vi "CCD bias dependent spectrum.vi"() -> ()   [LabVIEW 2012]
uses:
  <vilib>/Utility/file.llb/Read From Spreadsheet File (DBL).vi
  Instance           3 35Saved   CCD photon image_540_800_CR .vi
  Instance           4 35Saved   CCD photon image_540_800_CR .vi
  Instance           5 35Saved   CCD photon image_540_800_CR .vi
  Instance           8 35Saved   CCD photon image_540_800_CR .vi
  Instance          12 35Saved   CCD photon image_540_800_CR .vi
panel:
  in  "offset":dbl
  in  "gain":dbl=1.0
  out "Window 2":cluster{"Y":dbl[], "Y":dbl[]}[](graph)
  out "Window 1":cluster{"Y":dbl[], "Y":dbl[]}[](graph)
  in  "bias to":dbl=950.0
  in  "Bias from":dbl=550.0
  in  "Full Range":bool
  in  "Full Range":bool
  out "Save As":string
  in  "Save Matrix2":bool
  out "Save As":string
  in  "Save Matrix1":bool
  in  "select 2":bool
  in  "select":bool
  in  "next 2":bool
  in  "next":bool
  in  "previous 2":bool
  in  "previous":bool
  in  "Do it":bool
  out "?":path
  out "?":path
  out "pixnum":i32
  in  "?":bool
  in  "stop 2":bool
  in  "spc to":dbl=950.0
  in  "Spc From":dbl=550.0
  in  "?":bool
  out "MAX":dbl
  out "MIN":dbl
  out "X":sgl
  out "Y":sgl
  out "px":dbl
  out "px":dbl
  out "eV":dbl format="%#_4g"
  out "eV":dbl format="%#_4g"
  in  "To":dbl
  in  "From":dbl
  out "spc size":dbl=32.0
  out "eV":dbl format="%#_4g"
  out "eV":dbl format="%#_4g"
  in  "To":dbl
  in  "From":dbl
  out "px":dbl
  out "px":dbl
  in  "#2":bool
  # "Input File"
  # "2 Files"
  # "1 File"
  # "1st"
  # "2nd"
  # "Spectra Range"
  # "nm"
  # "to"
  # "nm"
  # "From"
  # "Bias Range"
  # "From"
  # "to"
  # "eV"
  # "eV"
  # "nm"
  # "# of Pixel"
  # "# of Spectra"
  # "nm"
  # "Offset"
  # "Gain"
  # "Active Window"
  # "#1"
  # "#2"
  # "Cosmic Ray Removal"
  # "NO"
  # "YES"
  # "Value"
  # "Position"
  # "nm"
  # "nm"
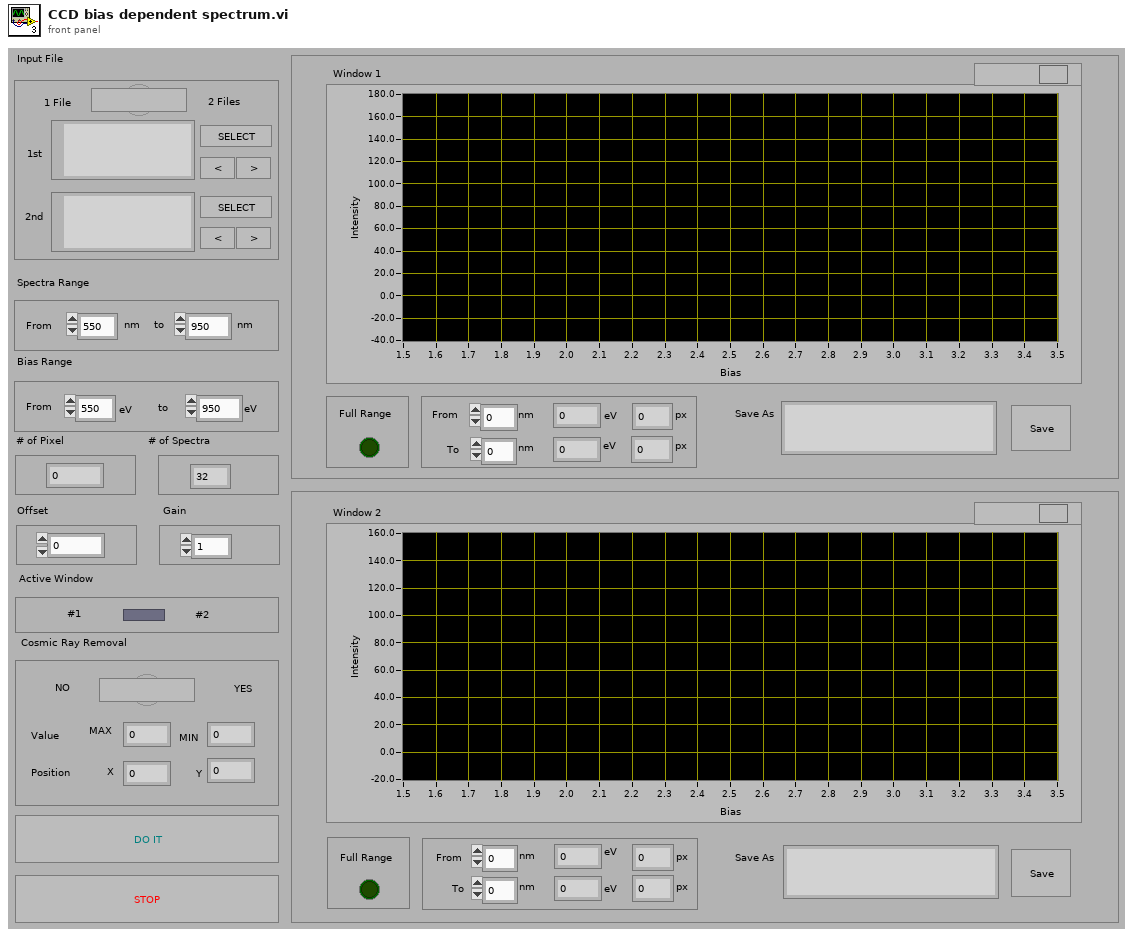
[diagram p1: front panel]
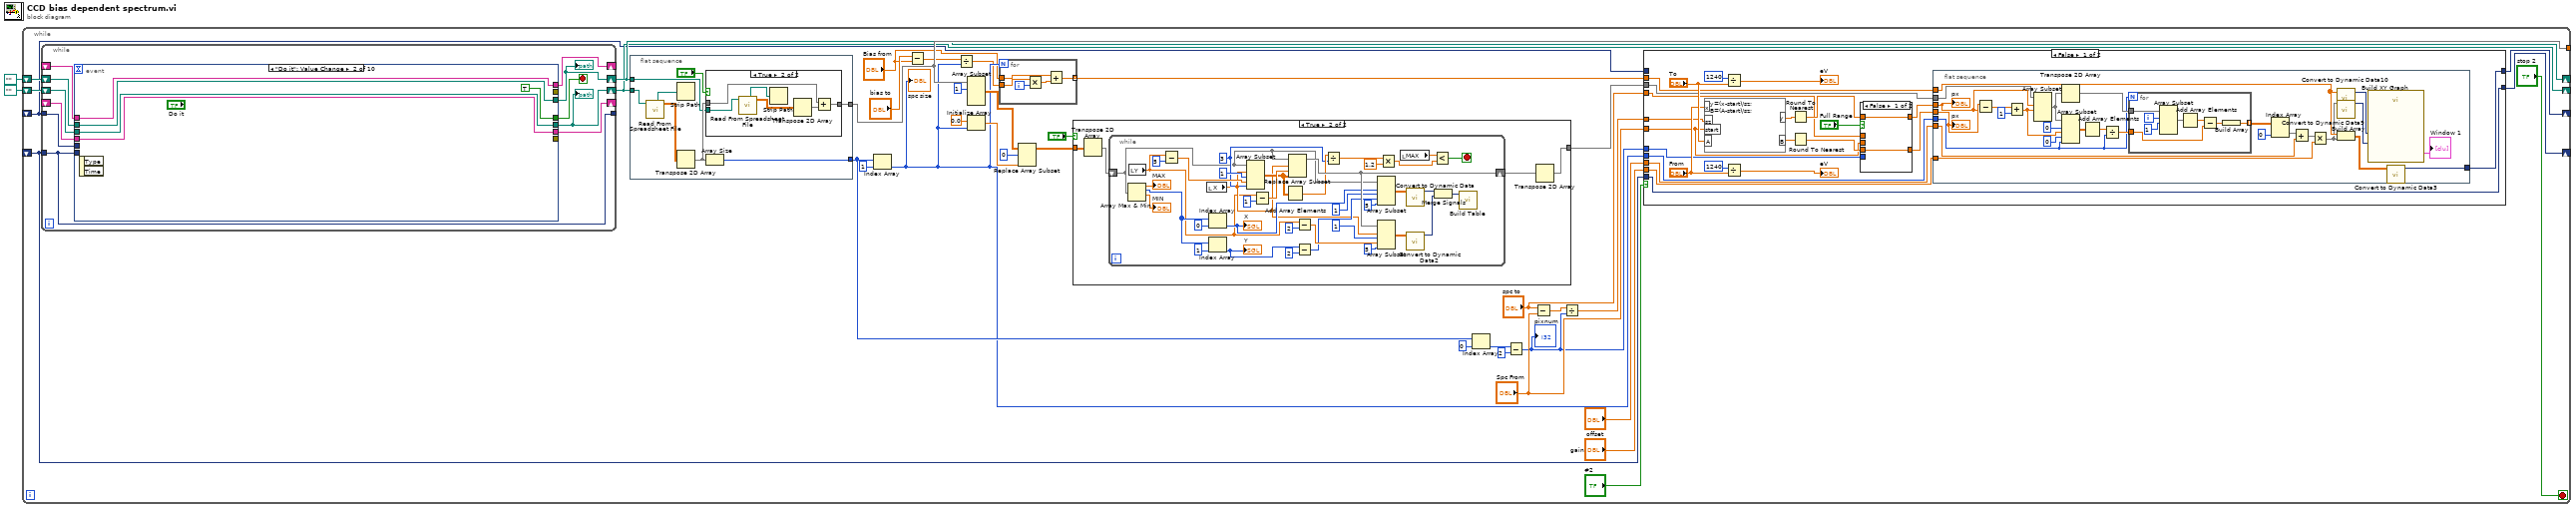
[diagram p0: block diagram]
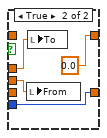
[diagram p2: hidden frame]
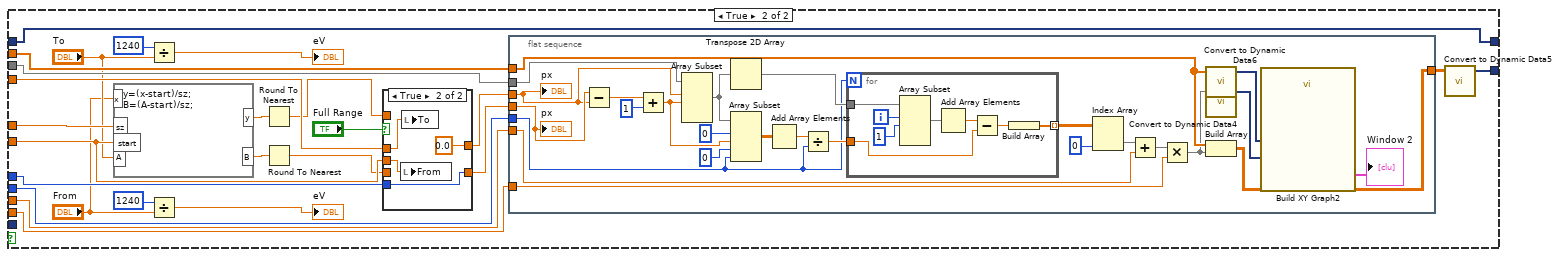
[diagram p3: hidden frame]
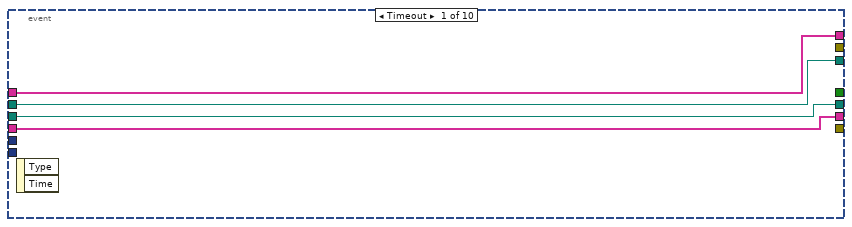
[diagram p5: hidden frame]
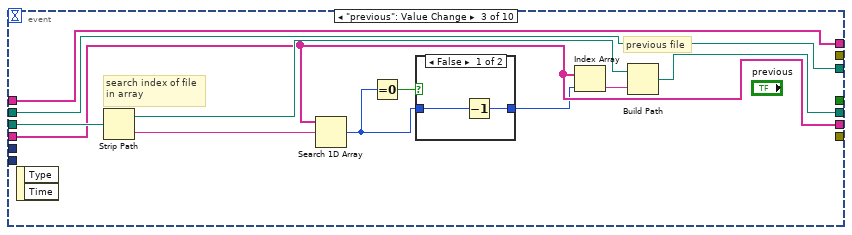
[diagram p6: hidden frame]
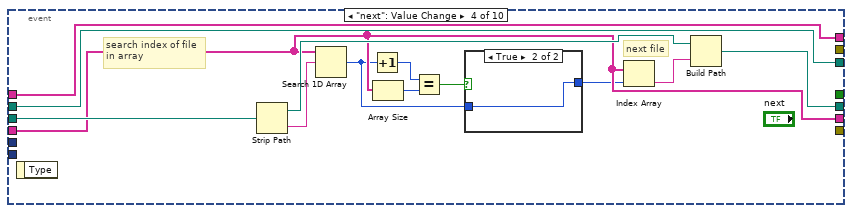
[diagram p8: hidden frame]
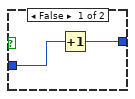
[diagram p9: hidden frame]
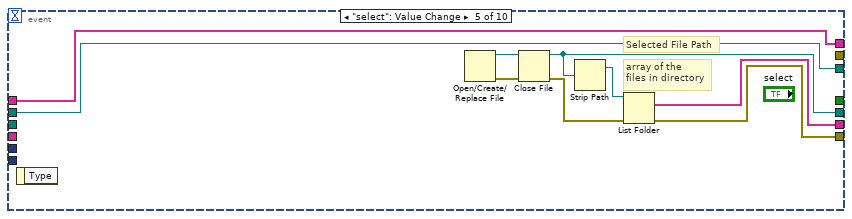
[diagram p10: hidden frame]
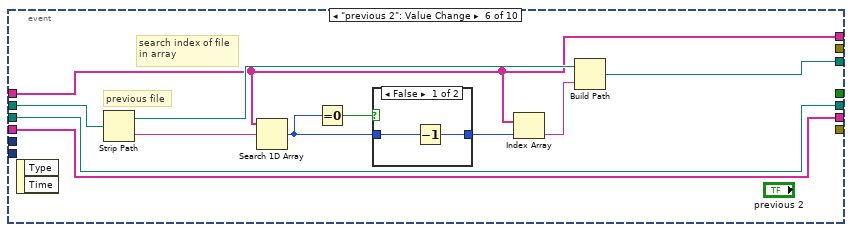
[diagram p11: hidden frame]
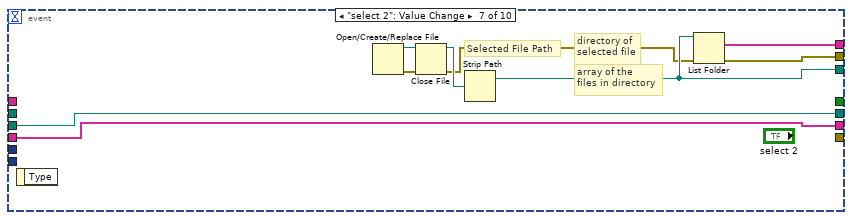
[diagram p13: hidden frame]
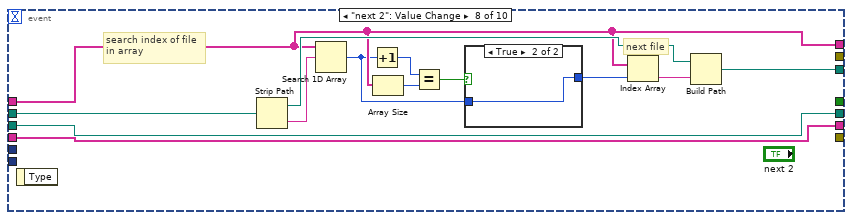
[diagram p14: hidden frame]
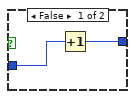
[diagram p15: hidden frame]
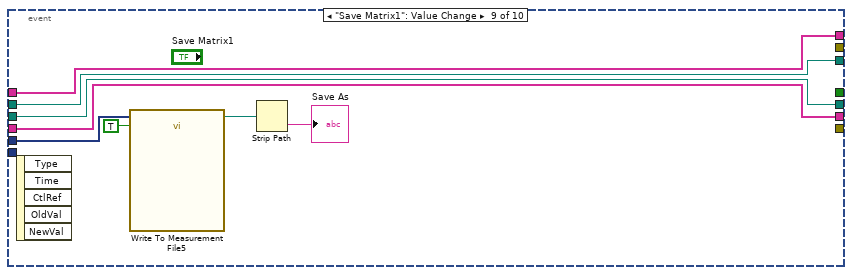
[diagram p16: hidden frame]
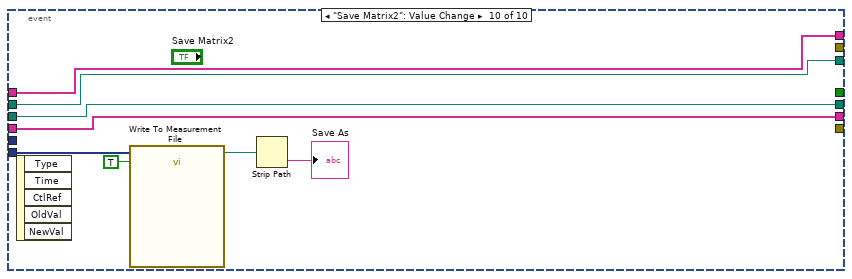
[diagram p17: hidden frame]
diagram:
  n1 = while {
    tunnel: [w27] -> _
    shift-right: [w20] -> _
    shift-left: path "" ("path") -> [w22]
    shift-right: [w21] -> _
    shift-left: path "" ("path") -> [w23]
    shift-right: [w19] -> _
    shift-left: _ -> [w5]
    shift-right: [w18] -> _
    shift-left: _ -> [w6]
    stop <- "stop 2" stop-if-true
    n2 = while {
      shift-right: [w185] -> _
      shift-left: _ -> [w184]
      shift-right: [w175] -> w20
      shift-left: w22 -> [w183]
      shift-right: [w176] -> w21
      shift-left: w23 -> [w182]
      shift-right: [w181] -> _
      shift-left: _ -> [w180]
      tunnel: w5 -> [w178]
      tunnel: w6 -> [w177]
      tunnel: [w177] -> _
      stop <- w179 stop-if-true
      n3 = event shown="[1] \"Do it\": Value Change" {
        selector: _ -> [_ _ _ _ _ _ _ _ _ _]
        dyn-events: _ -> [_ _ _ _ _ _ _ _ _ _]
        timeout: _ -> [_ _ _ _ _ _ _ _ _ _]
        tunnel: [_ TRUE _ _ _ _ _ _ _ _] -> w179
        tunnel: [w188 w193 w200 w218 w228 w234 w255 w264 w276 w282] -> w175
        tunnel: [w189 w194 w202 w214 w232 w239 w254 w263 w273 w281] -> w185
        tunnel: w184 -> [w189 w194 w202 w214 _ w239 w254 w263 w273 w281]
        tunnel: w183 -> [w188 w193 w205 w217 _ w234 w255 w264 w276 w282]
        tunnel: [w186 w191 w198 w215 w230 w235 w253 w265 w275 w283] -> w176
        tunnel: w182 -> [w186 w191 w198 w215 w230 w241 _ w266 w275 w283]
        tunnel: [w187 w192 w199 w216 w231 w240 w256 w259 w274 w284] -> w181
        tunnel: w180 -> [w187 w192 w199 w216 w231 w240 _ w259 w274 w284]
        tunnel: w178 -> [_ _ _ _ _ _ _ _ w280 _]
        tunnel: w177 -> [_ _ _ _ _ _ _ _ _ w288]
        tunnel: [_ _ _ _ _ _ w248 _ _ _] -> _
        tunnel: [_ _ _ _ w225 _ _ _ _ _] -> _
        event Timeout {
          n4 = event-data() -> ()  [unwired: 1 in, 2 out]
        }
        event "Do it": Value Change {
          n5 = event-data() -> ()  [unwired: 1 in, 2 out]
        }
        event "previous": Value Change {
          # "previous file"
          # "search index of file\nin array"
          n6 = event-data() -> ()  [unwired: 1 in, 2 out]
          n7 = Strip Path(path=w205) -> (stripped path=w203:path, name=w204:string)
          n8 = Search 1D Array(1D array=w202, element=w204) -> (index of element=w196:i32)  [unwired: 1 in]
          n9 = Equal To 0?(x=w196) -> (x = 0?=w197:bool)
          n10 = case shown="False" w197 {
            tunnel: w196 -> [w207 w208]
            tunnel: [w206 w208] -> w195
            frame False {
              n11 = Decrement(x=w207) -> (x-1=w206:i32)
            }
            frame True {
            }
          }
          n12 = Index Array(array=w202, index=w195) -> (element=w201:string)
          n13 = Build Path(base path=w203, name or relative path=w201) -> (appended path=w200:path)
        }
        event "next": Value Change {
          # "next file"
          # "search index of file\nin array"
          n14 = event-data() -> ()  [unwired: 1 in, 1 out]
          n15 = Strip Path(path=w217) -> (stripped path=w220:path, name=w221:string)
          n16 = Search 1D Array(1D array=w214, element=w221) -> (index of element=w209:i32)  [unwired: 1 in]
          n17 = Increment(x=w209) -> (x+1=w210:i32)
          n18 = Array Size(array=w214) -> (size(s)=w213:i32)
          n19 = Equal?(x=w210, y=w213) -> (x = y?=w212:bool)
          n20 = case shown="True" w212 {
            tunnel: w209 -> [w223 w224]
            tunnel: [w222 w224] -> w211
            frame False {
              n21 = Increment(x=w223) -> (x+1=w222:i32)
            }
            frame True {
            }
          }
          n22 = Index Array(array=w214, index=w211) -> (element=w219:string)
          n23 = Build Path(base path=w220, name or relative path=w219) -> (appended path=w218:path)
        }
        event "select": Value Change {
          # "array of the \nfiles in directory"
          # "Selected File Path"
          n24 = event-data() -> ()  [unwired: 1 in, 1 out]
          n25 = Open/Create/Replace File() -> (refnum out=w229:refnum<file>, error out=w227:errorcluster)  [unwired: 6 in, 1 out]
          n26 = Close File(refnum=w229, error in=w227) -> (path=w228:path, error out=w226:errorcluster)
          n27 = Strip Path(path=w228) -> (stripped path=w233:path)  [unwired: 1 out]
          n28 = List Folder(path=w233, error in=w226) -> (filenames=w232:string[], error out=w225:errorcluster)  [unwired: 2 in, 2 out]
        }
        event "previous 2": Value Change {
          # "previous file"
          # "search index of file\nin array"
          n29 = event-data() -> ()  [unwired: 1 in, 2 out]
          n30 = Strip Path(path=w241) -> (stripped path=w243:path, name=w244:string)
          n31 = Search 1D Array(1D array=w240, element=w244) -> (index of element=w237:i32)  [unwired: 1 in]
          n32 = Equal To 0?(x=w237) -> (x = 0?=w238:bool)
          n33 = case shown="False" w238 {
            tunnel: w237 -> [w246 w247]
            tunnel: [w245 w247] -> w236
            frame False {
              n34 = Decrement(x=w246) -> (x-1=w245:i32)
            }
            frame True {
            }
          }
          n35 = Index Array(array=w240, index=w236) -> (element=w242:string)
          n36 = Build Path(base path=w243, name or relative path=w242) -> (appended path=w235:path)
        }
        event "select 2": Value Change {
          # "array of the \nfiles in directory"
          # "directory of\nselected file"
          # "Selected File Path"
          n37 = event-data() -> ()  [unwired: 1 in, 1 out]
          n38 = Open/Create/Replace File() -> (refnum out=w252:refnum<file>, error out=w250:errorcluster)  [unwired: 6 in, 1 out]
          n39 = Close File(refnum=w252, error in=w250) -> (path=w251:path, error out=w249:errorcluster)
          n40 = Strip Path(path=w251) -> (stripped path=w253:path)  [unwired: 1 out]
          n41 = List Folder(path=w253, error in=w249) -> (filenames=w256:string[], error out=w248:errorcluster)  [unwired: 2 in, 2 out]
        }
        event "next 2": Value Change {
          # "next file"
          # "search index of file\nin array"
          n42 = event-data() -> ()  [unwired: 1 in, 1 out]
          n43 = Strip Path(path=w266) -> (stripped path=w268:path, name=w269:string)
          n44 = Search 1D Array(1D array=w259, element=w269) -> (index of element=w258:i32)  [unwired: 1 in]
          n45 = Increment(x=w258) -> (x+1=w260:i32)
          n46 = Array Size(array=w259) -> (size(s)=w262:i32)
          n47 = Equal?(x=w260, y=w262) -> (x = y?=w261:bool)
          n48 = case shown="True" w261 {
            tunnel: w258 -> [w271 w272]
            tunnel: [w270 w272] -> w257
            frame False {
              n49 = Increment(x=w271) -> (x+1=w270:i32)
            }
            frame True {
            }
          }
          n50 = Index Array(array=w259, index=w257) -> (element=w267:string)
          n51 = Build Path(base path=w268, name or relative path=w267) -> (appended path=w265:path)
        }
        event "Save Matrix1": Value Change {
          n52 = event-data() -> ()  [unwired: 1 in, 5 out]
          n53 = call "Write To Measurement File5"("Signals"=w280, "Reset"=TRUE) -> ("Filename Out"=w278:path)  [unwired: 15 in, 2 out]
          n54 = Strip Path(path=w278) -> (name=→"Save As":string)  [unwired: 1 out]
        }
        event "Save Matrix2": Value Change {
          n55 = event-data() -> ()  [unwired: 1 in, 5 out]
          n56 = call "Write To Measurement File"("Signals"=w288, "Reset"=TRUE) -> ("Filename Out"=w286:path)  [unwired: 15 in, 2 out]
          n57 = Strip Path(path=w286) -> (name=→"Save As":string)  [unwired: 1 out]
        }
      }
      "?" <- w175
      "?" <- w176
    }
    n58 = flat-sequence {
      tunnel: [w295] -> w27
      tunnel: [w292] -> w15
      tunnel: w20 -> [w290]
      tunnel: w21 -> [w289]
      frame #0 {
        n59 = call-poly <vilib>:"Read From Spreadsheet File.vi"("file path (dialog if empty)"=w290) -> ("all rows"=w293:dbl[][], "new file path (Not A Path if cancelled)"=w296:path)  [unwired: 6 in, 3 out]
        n60 = Strip Path(path=w296) -> ()  [unwired: 2 out]
        n61 = Transpose 2D Array(2D array=w293) -> (transposed array=w291:dbl[][])
        n62 = case shown="True" "?" {
          tunnel: w291 -> [w297 w302]
          tunnel: [w297 w301] -> w295
          tunnel: w289 -> [_ w298]
          frame False {
          }
          frame True {
            n63 = call-poly <vilib>:"Read From Spreadsheet File.vi"("file path (dialog if empty)"=w298) -> ("all rows"=w300:dbl[][], "new file path (Not A Path if cancelled)"=w303:path)  [unwired: 6 in, 3 out]
            n64 = Strip Path(path=w303) -> ()  [unwired: 2 out]
            n65 = Transpose 2D Array(2D array=w300) -> (transposed array=w299:dbl[][])
            n66 = Add(x=w302, y=w299) -> (x+y=w301:dbl[][])
          }
        }
        n67 = Array Size(array=w291) -> (size(s)=w292:i32[])
      }
    }
    n68 = Index Array(array=w15, index=1) -> (element=w11:i32)
    "spc size" <- w11
    n69 = Subtract(x="bias to", y="Bias from") -> (x-y=w12:dbl)
    n70 = Divide(x=w12, y=w11) -> (x/y=w10:dbl)
    n71 = Array Subset(array=w27, index (row)=1) -> (w36:dbl[][])  [unwired: 3 in]
    n72 = Initialize Array(0.0 ("element"), w11) -> (w38:dbl[])
    n73 = for {
      N: w11 -> [_]
      tunnel: [w170] -> w8 mode=indexing
      tunnel: w10 -> [w173]
      tunnel: "Bias from" -> [w171]
      i -> [w174]
      n74 = Multiply(x=w173, y=w174) -> (x*y=w172:dbl)
      n75 = Add(x=w171, y=w172) -> (x+y=w170:dbl)
    }
    n76 = Replace Array Subset(array=w36, new element=w38, index (row)=0) -> (w34:dbl[][])  [unwired: 1 in]
    n77 = case shown="True" "?" {
      tunnel: w34 -> [w304 w308]
      tunnel: [w304 w306] -> w33
      frame False {
      }
      frame True {
        n78 = Transpose 2D Array(2D array=w308) -> (transposed array=w307:dbl[][])
        n79 = while {
          shift-right: [w345] -> w305
          shift-left: w307 -> [w309]
          stop <- w324 stop-if-true
          w322 = 3
          n80 = Array Max & Min(array=w309) -> (max value=→"MAX":dbl, max index (indices)=w343:i32[], min value=→"MIN":dbl)  [unwired: 1 out]
          n81 = local read "Y"() -> (w311:sgl)
          n82 = Subtract(x=w311, y=5) -> (x-y=w339:sgl)
          n83 = local read "X"() -> (w312:sgl)
          n84 = Index Array(array=w343, index=0) -> (element=w316:i32)
          "X" <- w316
          n85 = Index Array(array=w343, index=1) -> (element=w315:i32)
          "Y" <- w315
          n86 = Array Subset(array=w309, index (row)=w312, length (row)=1, index (col)=w339, length (col)=w322) -> (w321:dbl[][])
          n87 = Subtract(x=w311, y=1) -> (x-y=w338:sgl)
          n88 = Add Array Elements(numeric array=w321) -> (sum=w323:dbl)
          n89 = Replace Array Subset(array=w309, new element=w321, index (row)=w312, index (col)=w338) -> (w345:dbl[][])
          n90 = Subtract(x=w311, y=2) -> (x-y=w334:sgl)
          n91 = Subtract(x=w315, y=2) -> (x-y=w329:i32)
          n92 = Divide(x=w323, y=w322) -> (x/y=w320:dbl)
          n93 = Array Subset(array=w309, index (row)=w316, length (row)=1, index (col)=w329, length (col)=5) -> (w327:dbl[][])
          n94 = Array Subset(array=w345, index (row)=w312, length (row)=1, index (col)=w334, length (col)=5) -> (w332:dbl[][])
          n95 = Multiply(x=w320, y=1.2) -> (x*y=w325:dbl)
          n96 = local read "MAX"() -> (w310:dbl)
          n97 = call "Convert to Dynamic Data"("2D Array"=w327) -> ("Dynamic Data Type"=w319:dynamicdata)  [unwired: 3 in]
          n98 = call "Convert to Dynamic Data2"("2D Array"=w332) -> ("Dynamic Data Type"=w317:dynamicdata)  [unwired: 3 in]
          n99 = Less?(x=w310, y=w325) -> (x < y?=w324:bool)
          n100 = Merge Signals(w319, w317) -> (w318:dynamicdata)
          n101 = call "Build Table"("Signals"=w318) -> ()  [unwired: 9 in, 2 out]
        }
        n102 = Transpose 2D Array(2D array=w305) -> (transposed array=w306:dbl[][])
      }
    }
    n103 = Index Array(array=w15, index=0) -> (element=w25:i32)
    n104 = Subtract(x=w25, y=2) -> (x-y=w17:i32)
    "pixnum" <- w17
    n105 = Subtract(x="spc to", y="Spc From") -> (x-y=w31:dbl)
    n106 = Divide(x=w31, y=w17) -> (x/y=w30:dbl)
    n107 = case shown="False" "#2" {
      tunnel: w11 -> [w55 w129]
      tunnel: w33 -> [w54 w128]
      tunnel: w30 -> [w53 w127]
      tunnel: "Spc From" -> [w45 w126]
      tunnel: [w52 w121] -> w19
      tunnel: [w42 w125] -> w18
      tunnel: w17 -> [w46 w123]
      tunnel: "spc to" -> [w44 w124]
      tunnel: w8 -> [w43 w122]
      tunnel: w6 -> [w42 _]
      tunnel: w5 -> [_ w121]
      tunnel: "offset" -> [w41 w120]
      tunnel: "gain" -> [w40 w119]
      frame False {
        n108 = formula code="y=(x-start)/sz;\nB=(A-start)/sz;"("x"="From", "A"="To", "sz"=w53, "start"=w45) -> ("y"=w57:dbl, "B"=w56:dbl)
        n109 = Divide(x=1240, y="To") -> (x/y=→"eV":dbl)
        n110 = Divide(x=1240, y="From") -> (x/y=→"eV":dbl)
        n111 = Round To Nearest(number=w57) -> (nearest integer value=w48:dbl)
        n112 = Round To Nearest(number=w56) -> (nearest integer value=w50:dbl)
        n113 = case shown="False" "Full Range" {
          tunnel: w50 -> [w65 _]
          tunnel: [w65 w66] -> w49
          tunnel: w48 -> [w64 _]
          tunnel: [w64 0.0] -> w47
          tunnel: w46 -> [_ w66]
          tunnel: w45 -> [_ w69]
          tunnel: w44 -> [_ w68]
          frame False {
          }
          frame True {
            n114 = local write "From"(w69) -> ()
            n115 = local write "To"(w68) -> ()
          }
        }
        n116 = flat-sequence {
          tunnel: [w96] -> w52
          tunnel: w49 -> [w93]
          tunnel: w47 -> [w92]
          tunnel: w55 -> [w82]
          tunnel: w54 -> [w85]
          tunnel: w43 -> [w76]
          tunnel: w41 -> [w74]
          tunnel: w40 -> [w71]
          frame #0 {
            n117 = Subtract(x=w93, y=w92) -> (x-y=w88:dbl)
            n118 = Add(x=w88, y=1) -> (x+y=w86:dbl)
            n119 = Array Subset(array=w85, index (row)=w92, length (row)=w86) -> (w84:dbl[][])  [unwired: 2 in]
            n120 = Transpose 2D Array(2D array=w84) -> (transposed array=w94:dbl[][])
            n121 = Array Subset(array=w84, index (row)=0, length (row)=w86, index (col)=0, length (col)=w82) -> (w83:dbl[][])
            n122 = Add Array Elements(numeric array=w83) -> (sum=w89:dbl)
            n123 = Divide(x=w89, y=w82) -> (x/y=w87:dbl)
            n124 = for {
              N: w82 -> [_]
              tunnel: w94 -> [w98]
              tunnel: [w100] -> w81 mode=indexing
              tunnel: w87 -> [w99]
              i -> [w104]
              n125 = Array Subset(array=w98, index (row)=w104, length (row)=1) -> (w97:dbl[][])  [unwired: 2 in]
              n126 = Add Array Elements(numeric array=w97) -> (sum=w102:dbl)
              n127 = Subtract(x=w102, y=w99) -> (x-y=w101:dbl)
              n128 = Build Array(w101) -> (w100:dbl[])
            }
            n129 = Index Array(array=w81, index (col)=0 ("disabled index (col)")) -> (element=w73:dbl[])  [unwired: 1 in]
            n130 = Add(x=w73, y=w74) -> (x+y=w72:dbl[])
            n131 = Multiply(x=w72, y=w71) -> (x*y=w70:dbl[])
            n132 = call "Convert to Dynamic Data10"("Array"=w76) -> ("Dynamic Data Type"=w78:dynamicdata)  [unwired: 3 in]
            n133 = call "Convert to Dynamic Data9"("Array"=w70) -> ("Dynamic Data Type"=w79:dynamicdata)  [unwired: 3 in]
            n134 = Build Array(w76, w70) -> (w75:dbl[][])
            n135 = call "Build XY Graph"("Y Input"=w79, "X Input"=w78) -> ("XY Graph"=→"Window 1":cluster{"Y":dbl[], "Y":dbl[]}[])  [unwired: 3 in, 6 out]
            n136 = call "Convert to Dynamic Data3"("2D Array"=w75) -> ("Dynamic Data Type"=w96:dynamicdata)  [unwired: 3 in]
            "px" <- w92
            "px" <- w93
          }
        }
      }
      frame True {
        n137 = formula code="y=(x-start)/sz;\nB=(A-start)/sz;"("x"="From", "A"="To", "sz"=w127, "start"=w126) -> ("y"=w112:dbl, "B"=w111:dbl)
        n138 = Divide(x=1240, y="To") -> (x/y=→"eV":dbl)
        n139 = Divide(x=1240, y="From") -> (x/y=→"eV":dbl)
        n140 = Round To Nearest(number=w112) -> (nearest integer value=w110:dbl)
        n141 = Round To Nearest(number=w111) -> (nearest integer value=w108:dbl)
        n142 = case shown="True" "Full Range" {
          tunnel: w108 -> [w131 _]
          tunnel: [w131 w134] -> w107
          tunnel: w110 -> [w130 _]
          tunnel: [w130 0.0] -> w109
          tunnel: w123 -> [_ w134]
          tunnel: w126 -> [_ w133]
          tunnel: w124 -> [_ w132]
          frame False {
          }
          frame True {
            n143 = local write "From"(w133) -> ()
            n144 = local write "To"(w132) -> ()
          }
        }
        n145 = flat-sequence {
          tunnel: w109 -> [w152]
          tunnel: w107 -> [w153]
          tunnel: w129 -> [w149]
          tunnel: w128 -> [w148]
          tunnel: w122 -> [w142]
          tunnel: [w141] -> w105
          tunnel: w120 -> [w137]
          tunnel: w119 -> [w136]
          frame #0 {
            n146 = Subtract(x=w153, y=w152) -> (x-y=w159:dbl)
            n147 = Add(x=w159, y=1) -> (x+y=w155:dbl)
            n148 = Array Subset(array=w148, index (row)=w152, length (row)=w155) -> (w151:dbl[][])  [unwired: 2 in]
            n149 = Transpose 2D Array(2D array=w151) -> (transposed array=w161:dbl[][])
            n150 = Array Subset(array=w151, index (row)=0, length (row)=w155, index (col)=0, length (col)=w149) -> (w150:dbl[][])
            n151 = Add Array Elements(numeric array=w150) -> (sum=w158:dbl)
            n152 = Divide(x=w158, y=w149) -> (x/y=w154:dbl)
            n153 = for {
              N: w149 -> [_]
              tunnel: w161 -> [w169]
              tunnel: [w162] -> w145 mode=indexing
              tunnel: w154 -> [w164]
              i -> [w168]
              n154 = Array Subset(array=w169, index (row)=w168, length (row)=1) -> (w167:dbl[][])  [unwired: 2 in]
              n155 = Add Array Elements(numeric array=w167) -> (sum=w165:dbl)
              n156 = Subtract(x=w165, y=w164) -> (x-y=w163:dbl)
              n157 = Build Array(w163) -> (w162:dbl[])
            }
            n158 = Index Array(array=w145, index (col)=0 ("disabled index (col)")) -> (element=w139:dbl[])  [unwired: 1 in]
            n159 = Add(x=w139, y=w137) -> (x+y=w140:dbl[])
            n160 = Multiply(x=w140, y=w136) -> (x*y=w138:dbl[])
            n161 = call "Convert to Dynamic Data6"("Array"=w142) -> ("Dynamic Data Type"=w146:dynamicdata)  [unwired: 3 in]
            n162 = call "Convert to Dynamic Data4"("Array"=w138) -> ("Dynamic Data Type"=w143:dynamicdata)  [unwired: 3 in]
            n163 = Build Array(w142, w138) -> (w141:dbl[][])
            n164 = call "Build XY Graph2"("Y Input"=w143, "X Input"=w146) -> ("XY Graph"=→"Window 2":cluster{"Y":dbl[], "Y":dbl[]}[])  [unwired: 3 in, 6 out]
            "px" <- w152
            "px" <- w153
          }
        }
        n165 = call "Convert to Dynamic Data5"("2D Array"=w105) -> ("Dynamic Data Type"=w125:dynamicdata)  [unwired: 3 in]
      }
    }
  }
